vi "checkArrSizeWithIdxArr.vi"(8 "error in (no error)":errorcluster, 9 "Idx Array":i32[](array[numeric]), 10 "Array Size":i32, 11 "MatOper in":refnum<class "MatOper.lvclass">) -> (0 "error out":errorcluster, 2 "In Spec":bool, 3 "MatOper out":refnum<class "MatOper.lvclass">)   [LabVIEW 2016, in "OfcFunc.lvlib" / "MatOper.lvclass"]
doc: "Check the element in index array is in the spec of array size or not."
uses:
  MatOper.lvclass
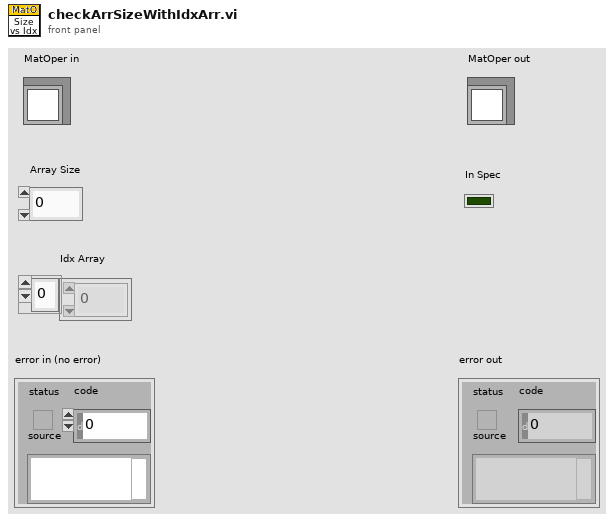
[diagram p1: front panel]
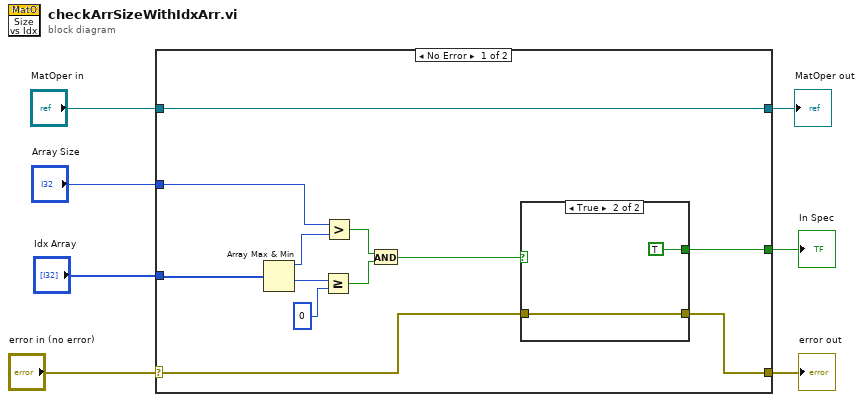
[diagram p0: block diagram]
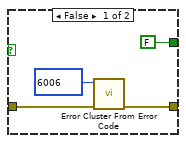
[diagram p2: hidden frame]
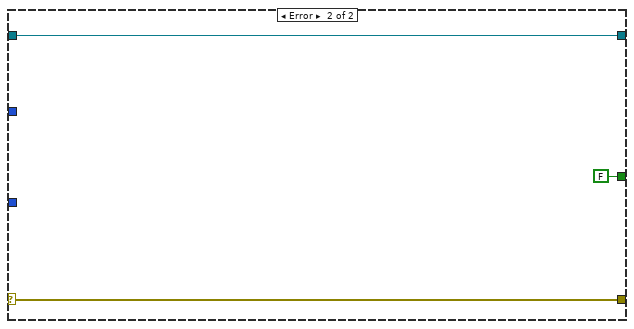
[diagram p3: hidden frame]
diagram:
  n1 = case shown="No Error" "error in (no error)" {
    selector: "error in (no error)" -> [w10 w28]
    tunnel: [w9 w28] -> w6
    tunnel: [w19 w27] -> w4
    tunnel: "MatOper in" -> [w19 w27]
    tunnel: "Array Size" -> [w12 _]
    tunnel: "Idx Array" -> [w11 _]
    tunnel: [w8 FALSE ("In Spec")] -> w1
    frame No Error {
      n2 = Array Max & Min(array=w11) -> (max value=w18:i32, min value=w17:i32)  [unwired: 2 out]
      n3 = Greater Or Equal?(x=w17, y=0) -> (x >= y?=w14:bool)
      n4 = Greater?(x=w12, y=w18) -> (0:w15:bool)
      n5 = And(x=w15, y=w14) -> (x .and. y?=w13:bool)
      n6 = case shown="True" w13 {
        tunnel: [FALSE ("In Spec") TRUE ("In Spec")] -> w8
        tunnel: w10 -> [w20 w24]
        tunnel: [w21 w24] -> w9
        frame False {
          n7 = call <vilib>:"Error Cluster From Error Code.vi"("error in (no error)"=w20, "error code (0)"=6006 ("code")) -> ("error out"=w21:errorcluster)  [unwired: 7 in]
        }
        frame True {
        }
      }
    }
    frame Error {
    }
  }
  "error out" <- w6
  "MatOper out" <- w4
  "In Spec" <- w1
